vi "Object Color detect.vi"() -> ()   [LabVIEW 2018]
doc: "Object Color Detection: This example is an example of object color detection, which can apply color space transformation for object tracking and extraction of objects with a specific color."
uses:
  vi.lib/VIRobotics/opencv_yiku/ctls/ColorConversionCodes.ctl
  vi.lib/VIRobotics/opencv_yiku/ctls/color.ctl
  vi.lib/VIRobotics/opencv_yiku/Mat/Mat_8U/Mat_8U.lvclass
  D:/Program Files/company/National Instruments/LabVIEW 2018/vi.lib/addons/VIRobotics/opencv_yiku/Mat/Mat/Mat.lvclass
  vi.lib/VIRobotics/opencv_yiku/Mat/Create_Mat_8U.vi
  vi.lib/VIRobotics/opencv_yiku/opencv_yiku.lvlib
  vi.lib/VIRobotics/opencv_yiku/Mat/Mat/Mat.lvclass
panel:
  out "img":picture
  out "res":picture
  out "edge":picture
  out "mask":picture
  # "Overview:  Demonstrates how to convert a BGR image to HSV, we can use this to extract a colored object.In our example, we will try to extract a red colored object.\nRequirements: Windows.\nInstructions: \n1. Run the VI"
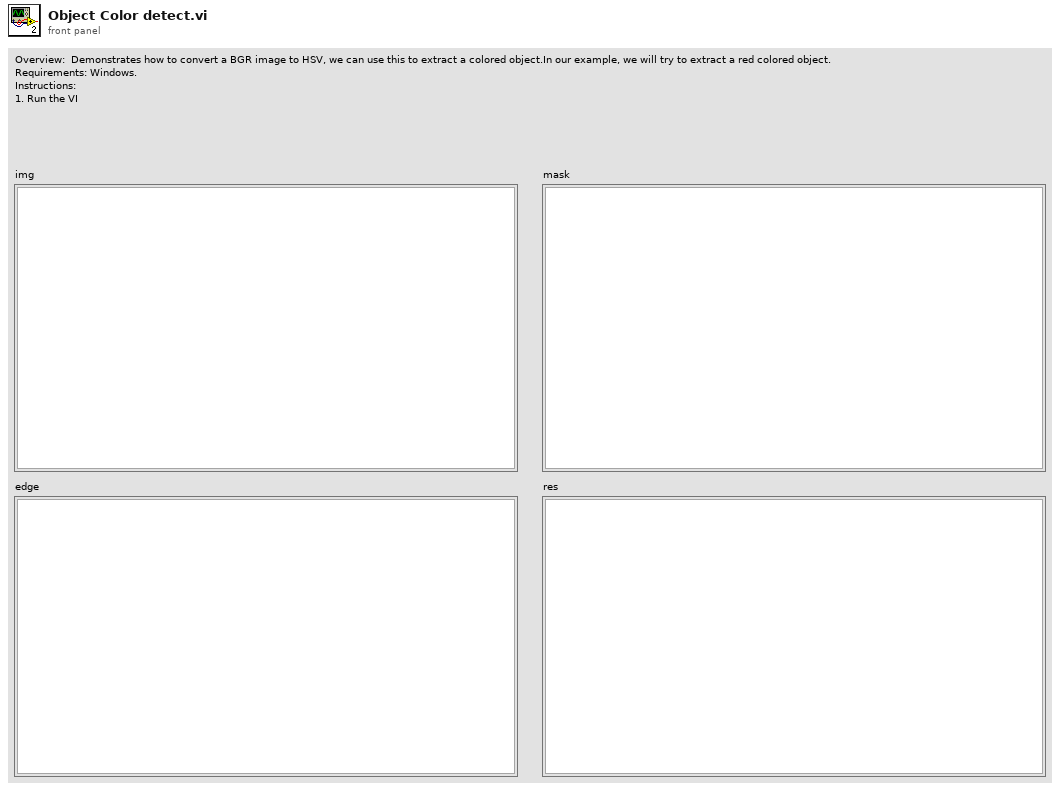
[diagram p1: front panel]
types:
  T1 = typedef "opencv_yiku.lvlib/ColorConversionCodes.ctl" = enum32{"COLOR_BGR2BGRA", "COLOR_BGRA2BGR", "COLOR_BGR2RGBA", "COLOR_RGBA2BGR", "COLOR_BGR2RGB", "COLOR_BGRA2RGBA", "COLOR_BGR2GRAY", "COLOR_RGB2GRAY", "COLOR_GRAY2BGR", "COLOR_GRAY2BGRA", "COLOR_BGRA2GRAY", "COLOR_RGBA2GRAY", "COLOR_BGR2BGR565", "COLOR_RGB2BGR565", "COLOR_BGR5652BGR", "COLOR_BGR5652RGB", "COLOR_BGRA2BGR565", "COLOR_RGBA2BGR565", "COLOR_BGR5652BGRA", "COLOR_BGR5652RGBA", "COLOR_GRAY2BGR565", "COLOR_BGR5652GRAY", "COLOR_BGR2BGR555", "COLOR_RGB2BGR555", "COLOR_BGR5552BGR", "COLOR_BGR5552RGB", "COLOR_BGRA2BGR555", "COLOR_RGBA2BGR555", "COLOR_BGR5552BGRA", "COLOR_BGR5552RGBA", "COLOR_GRAY2BGR555", "COLOR_BGR5552GRAY", "COLOR_BGR2XYZ", "COLOR_RGB2XYZ", "COLOR_XYZ2BGR", "COLOR_XYZ2RGB", "COLOR_BGR2YCrCb", "COLOR_RGB2YCrCb", "COLOR_YCrCb2BGR", "COLOR_YCrCb2RGB", "COLOR_BGR2HSV", "COLOR_RGB2HSV", "42", "43", "COLOR_BGR2Lab", "COLOR_RGB2Lab"}
  T2 = typedef "opencv_yiku.lvlib/color.ctl" = cluster{"c1":u8, "c2":u8, "c3":u8}
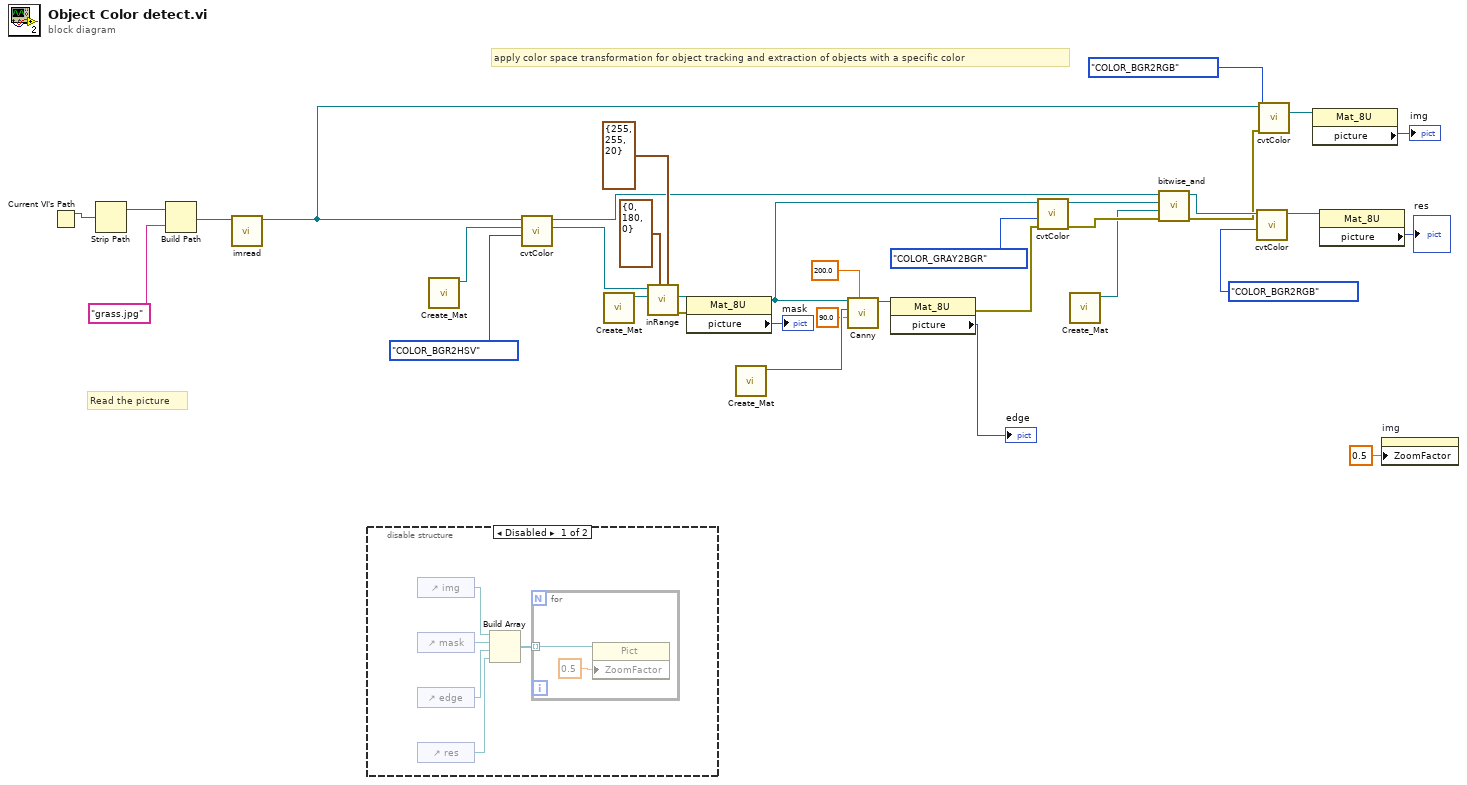
[diagram p0: block diagram]
diagram:
  # "apply color space transformation for object tracking and extraction of objects with a specific color"
  # "Read the picture"
  n1 = Current VI's Path() -> (path=w35:path)
  n2 = Strip Path(path=w35) -> (stripped path=w34:path)  [unwired: 1 out]
  n3 = Build Path(base path=w34, name or relative path="grass.jpg") -> (appended path=w32:path)
  n4 = call "imread.vi"("path"=w32) -> ("Mat out"=w4:refnum<class "Mat_8U.lvclass">)  [unwired: 9 in, 1 out]
  n5 = disable-structure shown="Disabled" {
    frame Disabled {
      n6 = control-ref of="img"() -> (w37:refnum<vi>)
      n7 = control-ref of="mask"() -> (w40:refnum<vi>)
      n8 = control-ref of="edge"() -> (w39:refnum<vi>)
      n9 = control-ref of="res"() -> (w36:refnum<vi>)
      n10 = Build Array(w37, w40, w39, w36) -> (w38:refnum<vi>[])
      n11 = for {
        tunnel: w38 -> [w42] mode=indexing
        n12 = property class="Pict"(reference=w42, "ZoomFactor"=sgl 0.5 ("Zoom Factor")) -> ()  [unwired: 1 in, 2 out]
      }
    }
    frame Enabled {
    }
  }
  n13 = call-poly "Create_Mat.vi"() -> ("Mat_8U_out"=w31:refnum<class "Mat_8U.lvclass">)  [unwired: 10 in, 1 out]
  n14 = call "cvtColor.vi"("dstCn"=ColorConversionCodes."COLOR_BGR2HSV", "dst"=w31, "src"=w4) -> ("dst out"=w29:refnum<class "Mat_8U.lvclass">, "src out"=w8:refnum<class "Mat_8U.lvclass">)  [unwired: 6 in, 1 out]
  n15 = call-poly "Create_Mat.vi"() -> ("Mat_8U_out"=w26:refnum<class "Mat_8U.lvclass">)  [unwired: 10 in, 1 out]
  n16 = call "inRange.vi"("higherb"=T2 {"c1"=255, "c2"=255, "c3"=20}, "lowerb"=T2 {"c1"=0, "c2"=180, "c3"=0}, "dst"=w26, "Mat"=w29) -> ("error out"=w25:errorcluster, "dst out"=w24:refnum<class "Mat_8U.lvclass">)  [unwired: 5 in, 1 out]
  n17 = property class="Mat_8U"(reference=w24, error in=w25) -> (reference out=w16:refnum<class "Mat_8U.lvclass">, "picture"=→"mask":picture)  [unwired: 1 out]
  n18 = call-poly "Create_Mat.vi"() -> ("Mat_8U_out"=w22:refnum<class "Mat_8U.lvclass">)  [unwired: 10 in, 1 out]
  n19 = call "Canny.vi"("threshold2"=200.0, "threshold1"=90.0, "dst in"=w22, "Mat in"=w16) -> ("dst out"=w19:refnum<class "Mat_8U.lvclass">)  [unwired: 6 in, 1 out]
  n20 = property class="Mat_8U"(reference=w19) -> (error out=w15:errorcluster, "picture"=→"edge":picture)  [unwired: 1 in, 1 out]
  n21 = call "cvtColor.vi"("error in (no error)"=w15, "dstCn"=ColorConversionCodes."COLOR_GRAY2BGR", "src"=w16) -> ("error out"=w14:errorcluster, "src out"=w11:refnum<class "Mat_8U.lvclass">)  [unwired: 6 in, 1 out]
  n22 = call-poly "Create_Mat.vi"() -> ("Mat_8U_out"=w13:refnum<class "Mat_8U.lvclass">)  [unwired: 10 in, 1 out]
  n23 = call "bitwise_and.vi"("error in (no error)"=w14, "dst"=w13, "src2"=w11, "src1"=w8) -> ("error out"=w2:errorcluster, "dst out"=w3:refnum<class "Mat_8U.lvclass">)  [unwired: 6 in]
  n24 = call "cvtColor.vi"("dstCn"=ColorConversionCodes."COLOR_BGR2RGB", "src"=w3) -> ("src out"=w10:refnum<class "Mat_8U.lvclass">)  [unwired: 7 in, 2 out]
  n25 = call "cvtColor.vi"("error in (no error)"=w2, "dstCn"=ColorConversionCodes."COLOR_BGR2RGB", "src"=w4) -> ("dst out"=w5:refnum<class "Mat_8U.lvclass">)  [unwired: 6 in, 2 out]
  n26 = property class="Mat_8U"(reference=w5) -> ("picture"=→"img":picture)  [unwired: 1 in, 2 out]
  n27 = property class="Mat_8U"(reference=w10) -> ("picture"=→"res":picture)  [unwired: 1 in, 2 out]
  n28 = property on="img" class="Pict"("ZoomFactor"=sgl 0.5 ("Zoom Factor")) -> ()  [unwired: 2 in, 2 out]
